vi "disconnect.vi"(8 "error in (no error)":errorcluster, 11 "SerialClient in":refnum<class "SerialCommunication.lvclass">) -> (0 "error out":errorcluster, 3 "SerialClient out":refnum<class "SerialCommunication.lvclass">)   [LabVIEW 2016, in "SerialCommunication.lvclass"]
uses:
  SerialCommunication.lvclass
  SerialCommunication.lvclass/SerialCommunication.ctl
  common_serialprotocols/SerialCommunicator/SerialCommunicator.lvclass
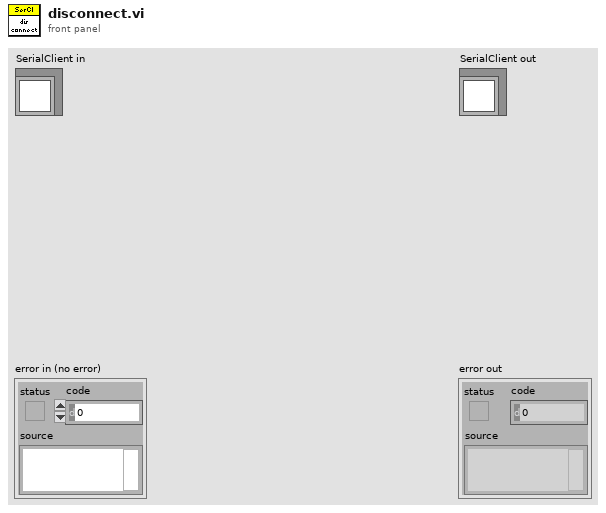
[diagram p1: front panel]
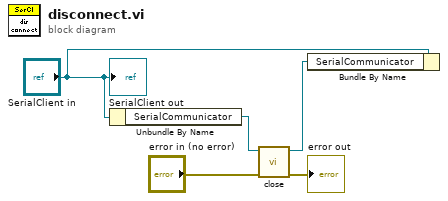
[diagram p0: block diagram]
diagram:
  n1 = Unbundle By Name("SerialClient in") -> ("SerialCommunicator"=w1:refnum<class "SerialCommunicator.lvclass">)
  n2 = call-dynamic "close.vi"("error in (no error)"="error in (no error)", "SerialCommunicator in"=w1) -> ("error out"=→"error out":errorcluster, "SerialCommunicator out"=w3:refnum<class "SerialCommunicator.lvclass">)  [unwired: 8 in]
  n3 = Bundle By Name(cluster="SerialClient in", "SerialCommunicator"=w3) -> ()  [unwired: 1 out]
  "SerialClient out" <- "SerialClient in"
